vi "read_attributes.vi"(8 "error in (no error)":errorcluster, 11 "SpectralClustering in":refnum<class "SpectralClustering.lvclass">) -> (0 "error out":errorcluster, 2 "attributes":T1, 3 "SpectralClustering out":refnum<class "SpectralClustering.lvclass">)   [LabVIEW 2020, in "SpectralClustering.lvclass"]
uses:
  SpectralClustering.lvclass
  Controls/spectral_clustering_attributes.ctl
  SpectralClustering.lvclass/SpectralClustering.ctl
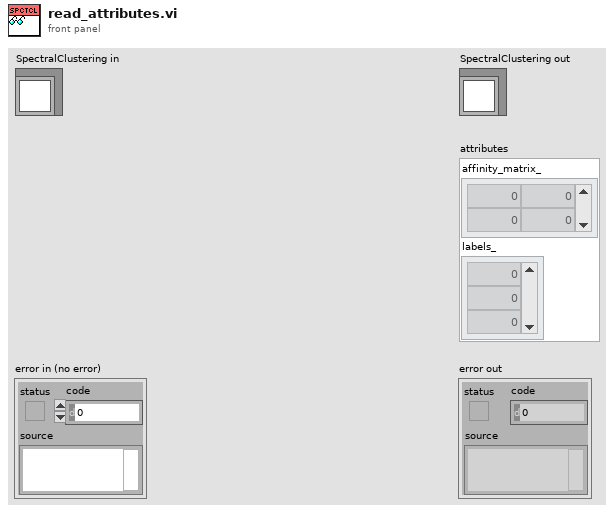
[diagram p1: front panel]
types:
  T1 = typedef "spectral_clustering_attributes.ctl" = cluster{"affinity_matrix_":dbl[][], "labels_":dbl[]}
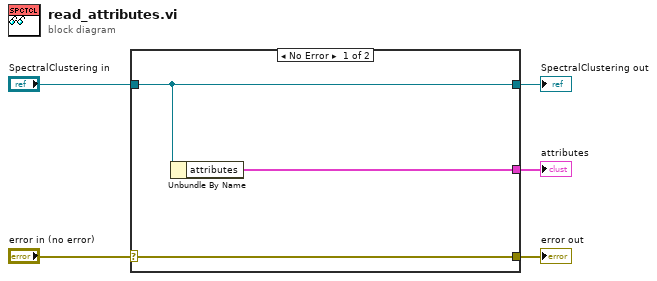
[diagram p0: block diagram]
diagram:
  n1 = case shown="No Error" "error in (no error)" {
    selector: "error in (no error)" -> [w8 w9]
    tunnel: [w8 w9] -> w4
    tunnel: [w7 w10] -> w2
    tunnel: "SpectralClustering in" -> [w7 w10]
    tunnel: [w6 _] -> w1
    frame No Error {
      n2 = Unbundle By Name(w7) -> ("attributes"=w6:T1)
    }
    frame Error {
    }
  }
  "error out" <- w4
  "SpectralClustering out" <- w2
  "attributes" <- w1
